vi "Time Since RE.vi"(1 "Input":bool) -> (0 "Time Since RE of Input":u32)   [LabVIEW 2013]
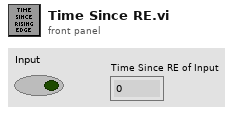
[diagram p1: front panel]
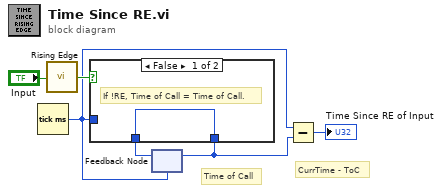
[diagram p0: block diagram]
diagram:
  # "Time of Call"
  # "CurrTime - ToC"
  n1 = Tick Count (ms)() -> (millisecond timer value=w2:u32)
  n2 = call "Rising Edge.vi"("Input"="Input") -> ("Rising Edge"=w4:bool)
  n3 = feedback #1(w2) -> (w1:u32)
  n4 = case shown="False" w4 {
    tunnel: w2 -> [_ w8]
    tunnel: [w7 w8] -> w3
    tunnel: w1 -> [w7 _]
    frame False {
      # "If !RE, Time of Call = Time of Call."
    }
    frame True {
      # "If RE, Time of Call = Time"
    }
  }
  n5 = feedback-in #1(w3) -> ()
  n6 = Subtract(x=w2, y=w1) -> (x-y=→"Time Since RE of Input":u32)
